vi "001_TCPTransfer.vi"(11 "Queue Ref":T1={"UI"=refnum, "Message"=refnum, "Data"=refnum, "Caller"=refnum, "Name"="000 Common", "Data Path"=path "D:/NBT/01-Project/02-Processing/NBT-TestPlatform V2/NBT-TestPlatform V2.0.3/Config/NBT/NBT_V1.0.0/Project/0001_HZKD_ST01/00_DataSource/001_PLC/01_PLC", "Class Path"=path "", "SubPanel"=refnum, "Project Name"="", "MNT"="", "Title"="", "Data Source"=refnum, "Queue List"={}, "VI"=refnum, "UE"=refnum}) -> ()   [LabVIEW 2020]
doc: "TCP"
uses:
  Alin/QMH/000 Module Data Type.ctl
  Alin/QMH/Queue Message.ctl
  9999 SubVI/Global/Data Global/SDQ Data Type.ctl
  0007 Controls/005 Data Source Type.ctl
  9999 SubVI/Global/Data Global/Data Global Mode.ctl
  9cf45a25-2d87-4abb-9e44-08fab8a6d34b.vi
panel:
  out "Status":bool
  in  "Port":u16=9090
  in  "Open":bool
  in  "Panel Show":bool
  out "Write Data":string
  out "Read Data":string
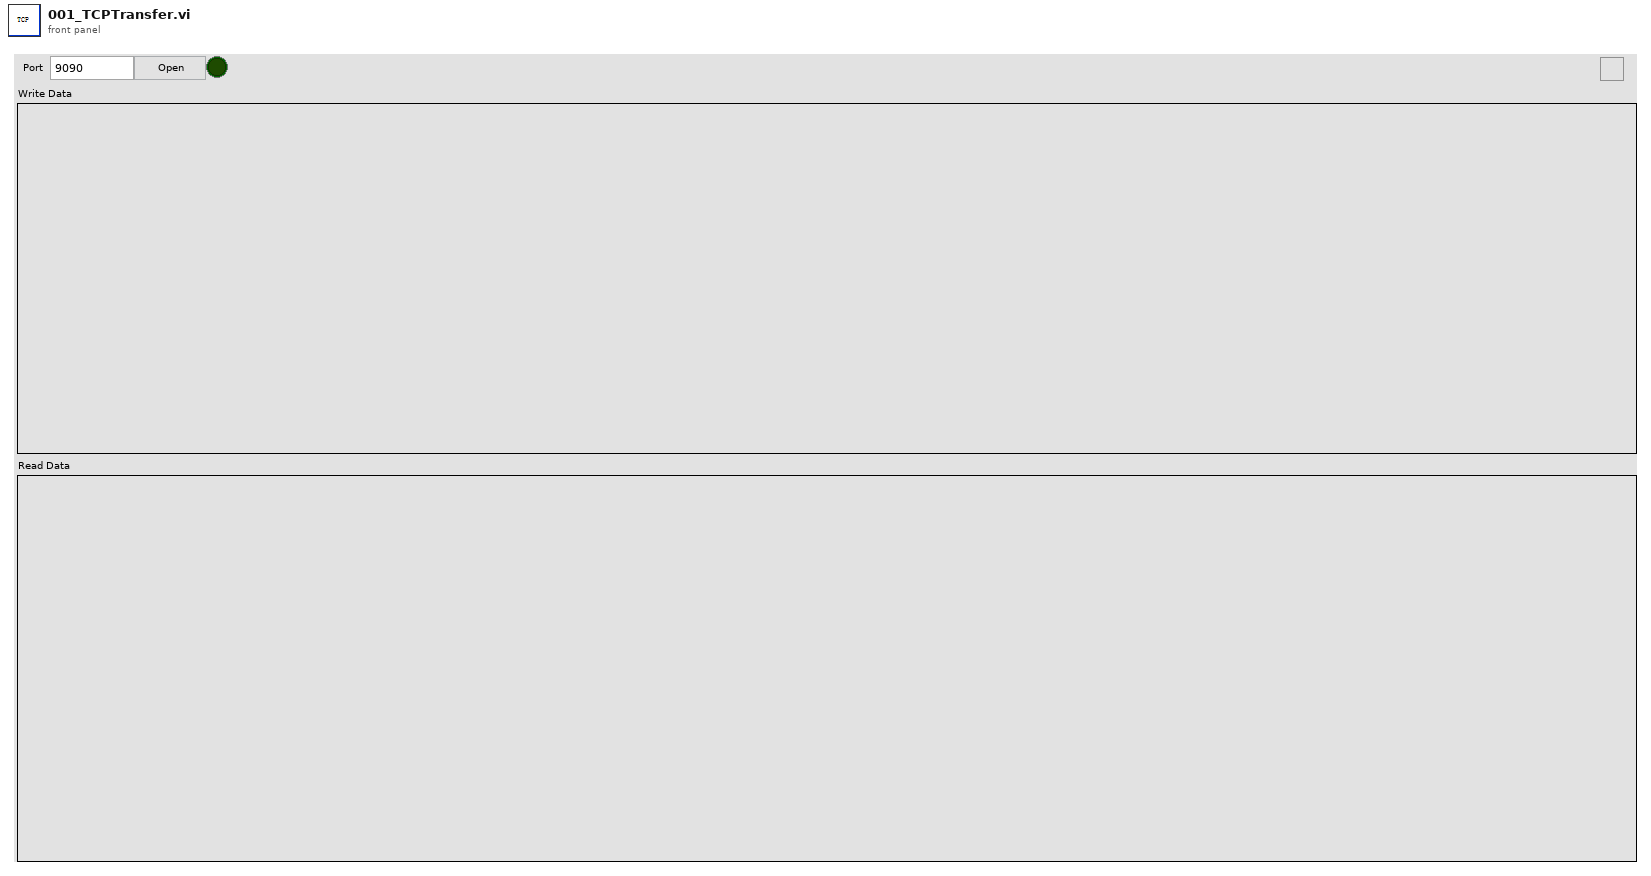
[diagram p1: front panel]
types:
  T1 = typedef "000 Module Data Type.ctl" = cluster{"UI":refnum<queue>, "Message":refnum<queue>, "Data":refnum<queue>, "Caller":refnum<queue>, "Name":string, "Data Path":path, "Class Path":path, "SubPanel":refnum<vi>, "Project Name":string, "MNT":string, "Title":string, "Data Source":refnum<queue>, "Queue List":map{string, refnum<queue>}, "VI":refnum<vi>, "UE":refnum<user-event>}
  T2 = typedef "SDQ Data Type.ctl" = cluster{"CAN Length":string, "CAN Name":string, "CAN ID":string, "CAN Type":string, "Test Item":string, "Byte Order":string, "Instruction":string, "Control Type":string, "Group":string, "Offset":dbl, "Coefficient":dbl, "Write Enable":bool, "Lable Type":string, "Key?":string, "Set Value":string, "Upper":dbl, "Lower":dbl, "Unit":string, "Formula":string, "Test Item Type":string, "Length":i32, "Address":string, "Name":string, "Identifier":string, "Data Type":string, "Enumerate?":string, "Enumerate List":string, "Data":string, "Source":string}
  T3 = typedef "005 Data Source Type.ctl" = cluster{"Device Name":string, "Device Model":string, "Device Driver":string, "IP Address":string, "Port":string, "Remark":string, "Enable":string, "Path":string}
  T4 = cluster{"Read Data":map{string, string}, "Open?":bool, "Start?":bool, "Queue Ref":T1, "Data":map{string, T2}, "Data List":T2[], "Ref":cluster{"Server":refnum<k5>, "Client":refnum<k5>}, "Identifiers":string, "Last Time":u32, "All Data":string[][], "Element":T2, "Title":string[], "Type":map{string, string}, "IP":string, "port":i32, "Next":string, "Data Type Out":T3, "Delay":cluster{"Count Time(ms)":u32, "Delay Time(ms)":u32, "Next":string}}
  T5 = typedef "Data Global Mode.ctl" = enum16{"Init", "Read", "Write", "Write Data", "Load"}
  T6 = cluster{"Server":refnum<k5>, "Client":refnum<k5>}
  T7 = cluster{"Name":string, "Type":map{string, string}}
  T8 = typedef "eventvkey.ctl" = enum16{"ASCII", "Enter", "Return", "Shift", "Ctrl", "Alt", "Cmd", "Opt", "Caps", "NumLock", "Clear", "Break", "Up", "Down", "Left", "Right", "Insert", "Delete", "Home", "End", "PageUp", "PageDown", "Escape", "Help", "Pause", "ScrollLock", "F1", "F2", "F3", "F4", "F5", "F6", "F7", "F8", "F9", "F10", "F11", "F12", "F13", "F14", "F15", "F16", "F17", "F18", "F19", "F20", "F21", "F22", "F23", "F24", "Play", "VolumeUp", "VolumeDown", "Mute", "Two Byte Char"}
  T9 = cluster{"Shift":bool, "Ctrl":bool, "Alt":bool, "Cmd":bool, "Opt":bool}
  T10 = cluster{"Queue List":map{string, refnum<queue>}, "Active Panel":string, "Queue":T1, "Active Row":i32, "All Data":string[][]}
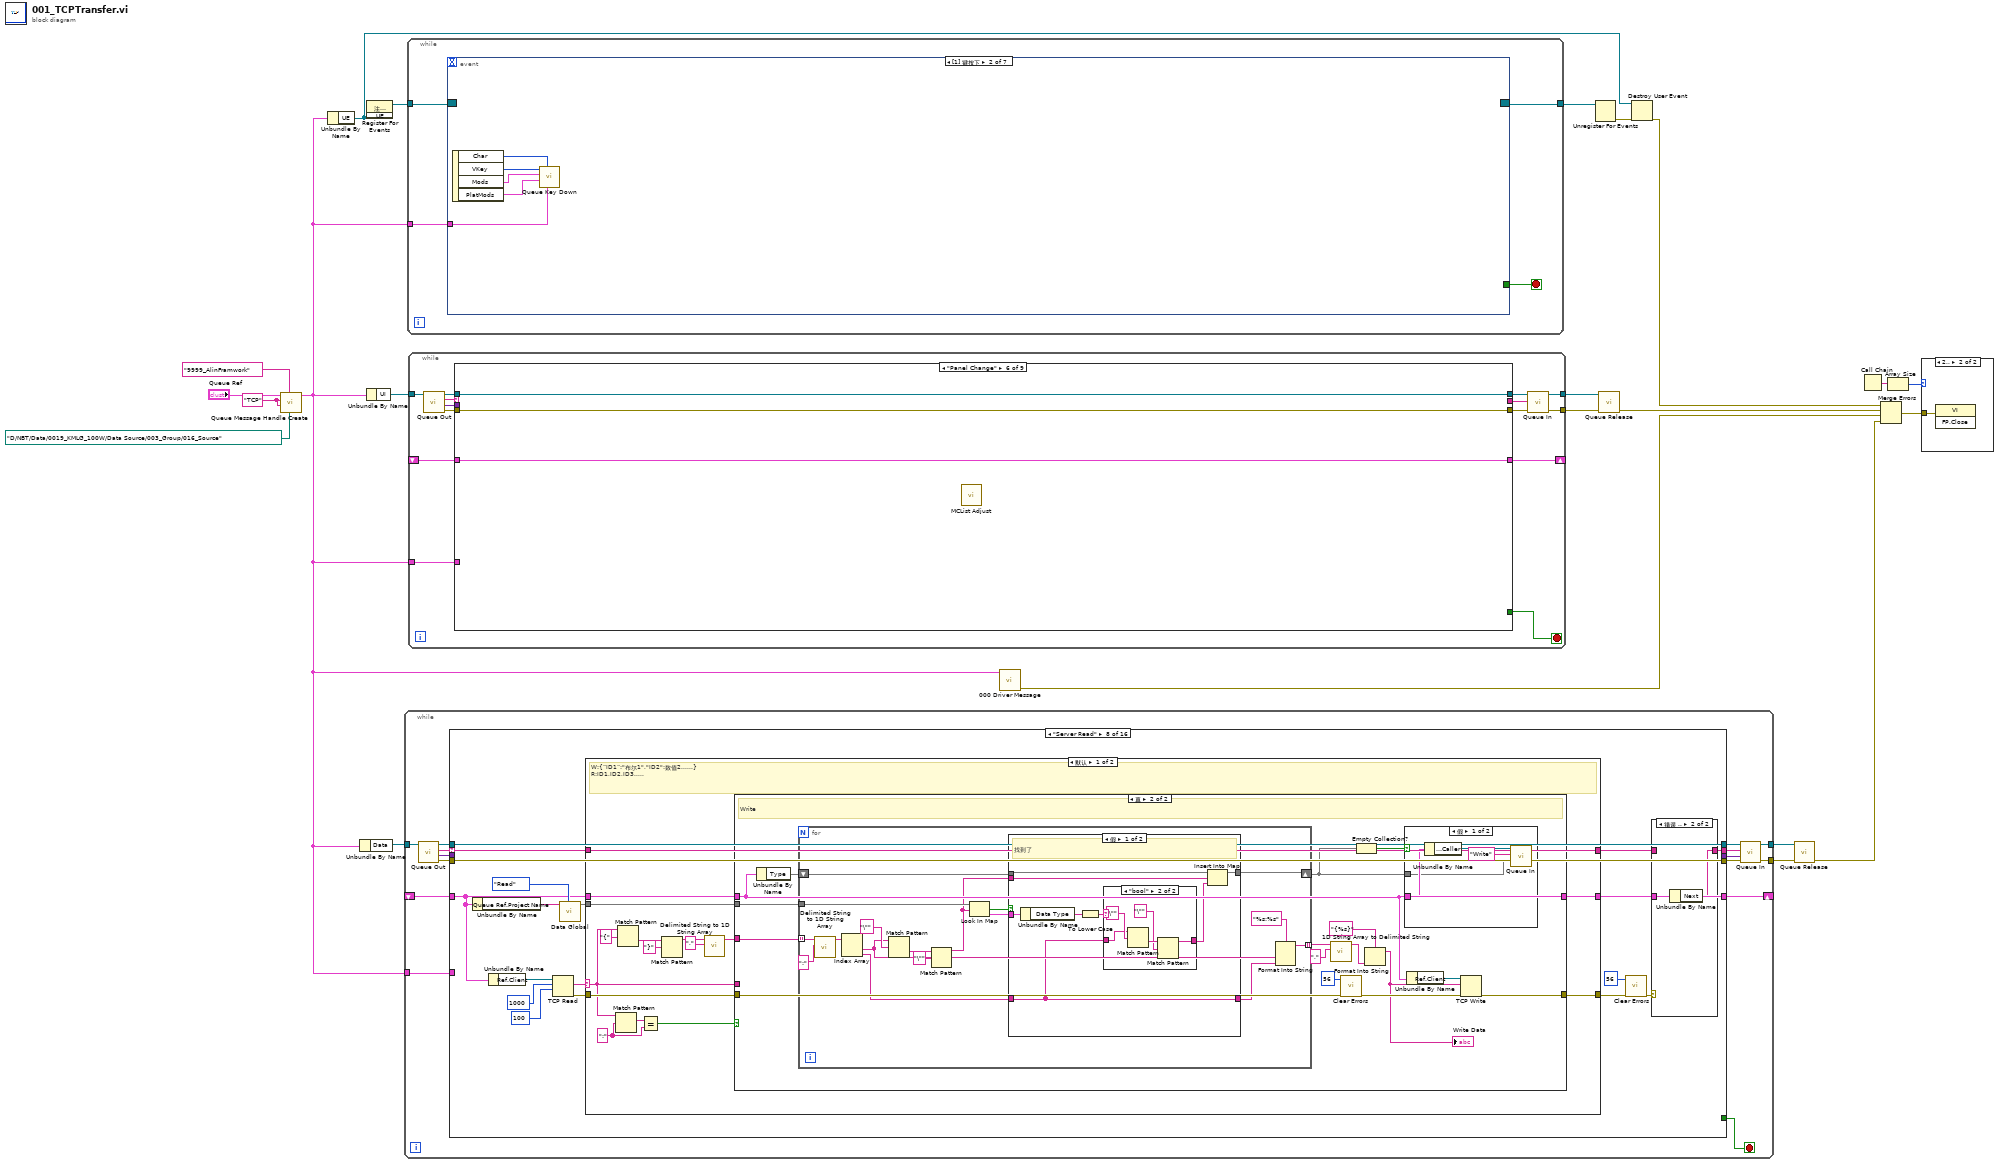
[diagram p0: block diagram]
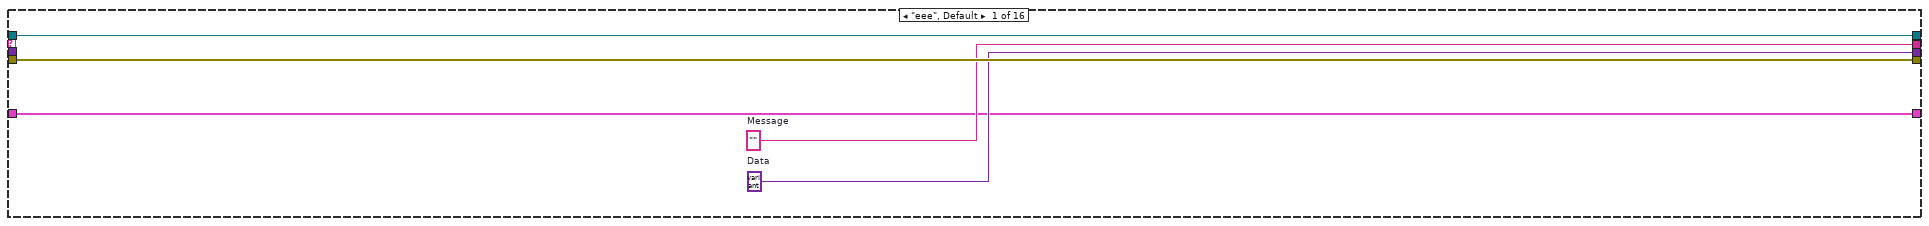
[diagram p2: hidden frame]
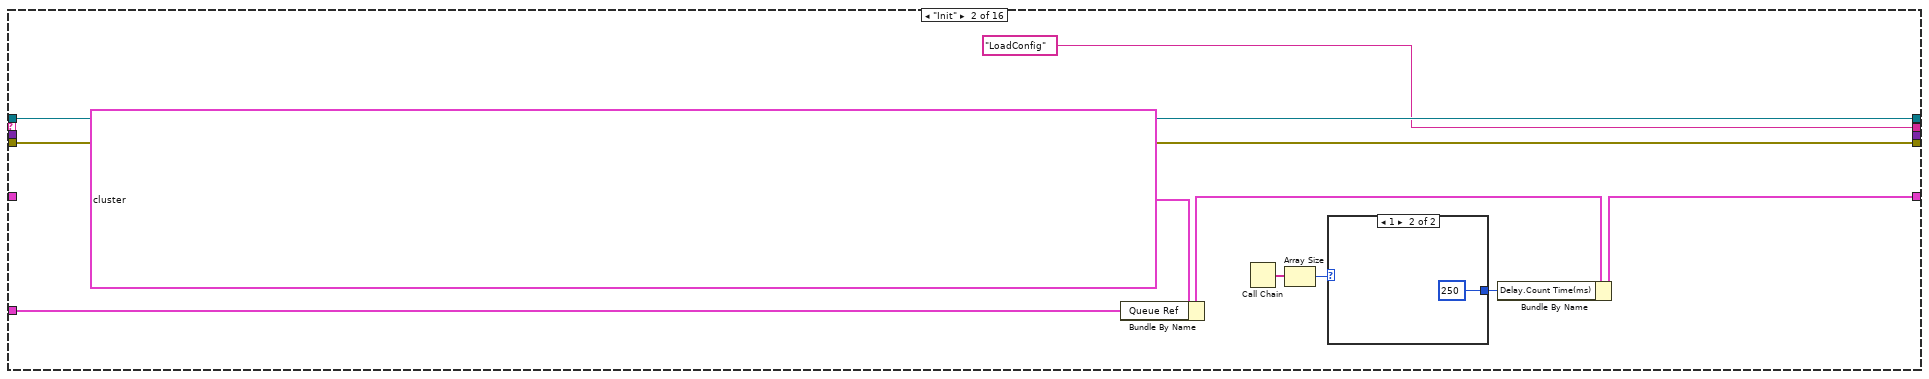
[diagram p3: hidden frame]
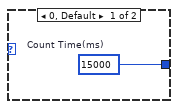
[diagram p4: hidden frame]
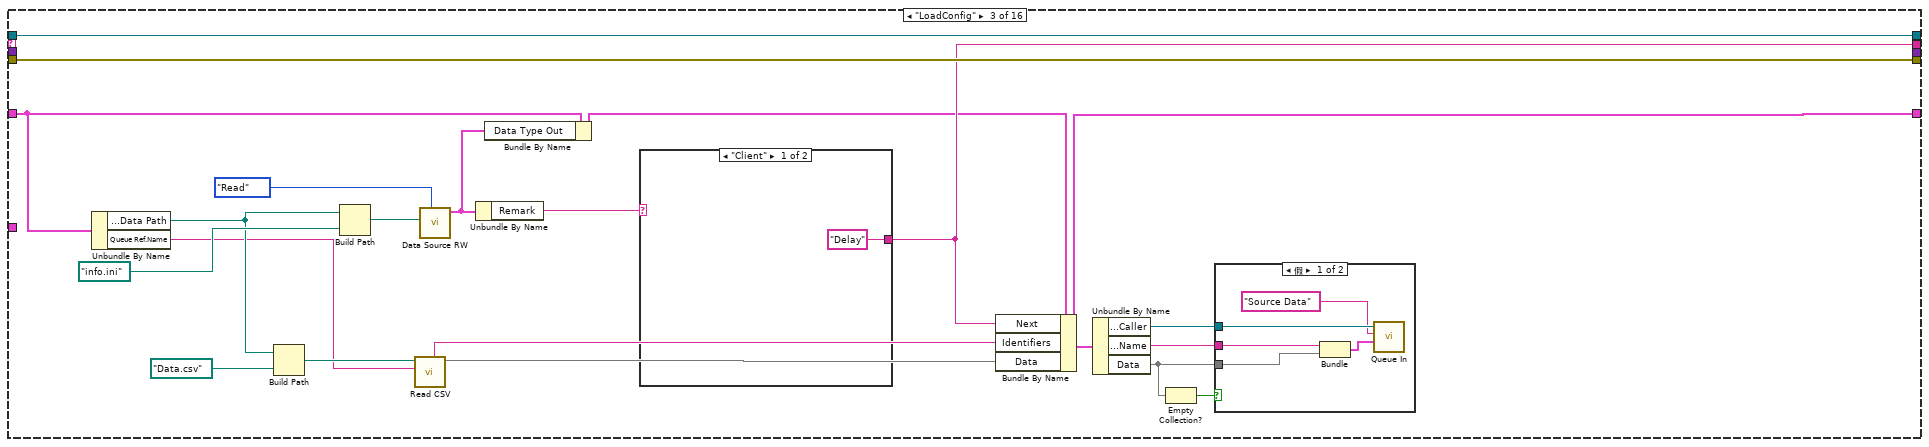
[diagram p5: hidden frame]
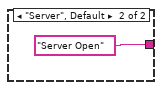
[diagram p7: hidden frame]
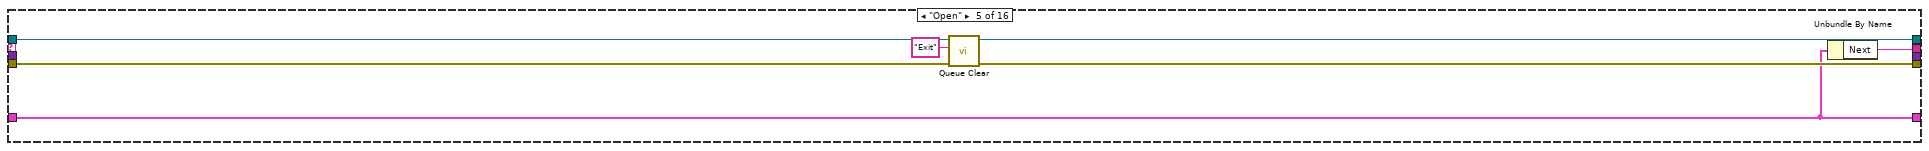
[diagram p9: hidden frame]
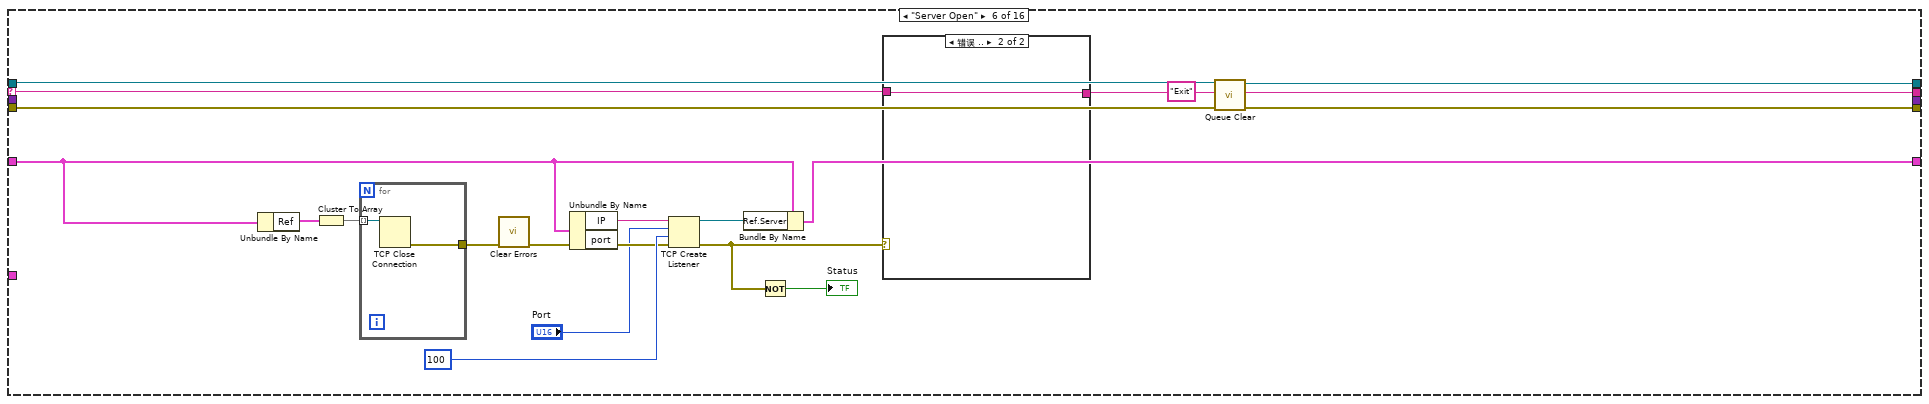
[diagram p10: hidden frame]
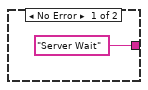
[diagram p11: hidden frame]
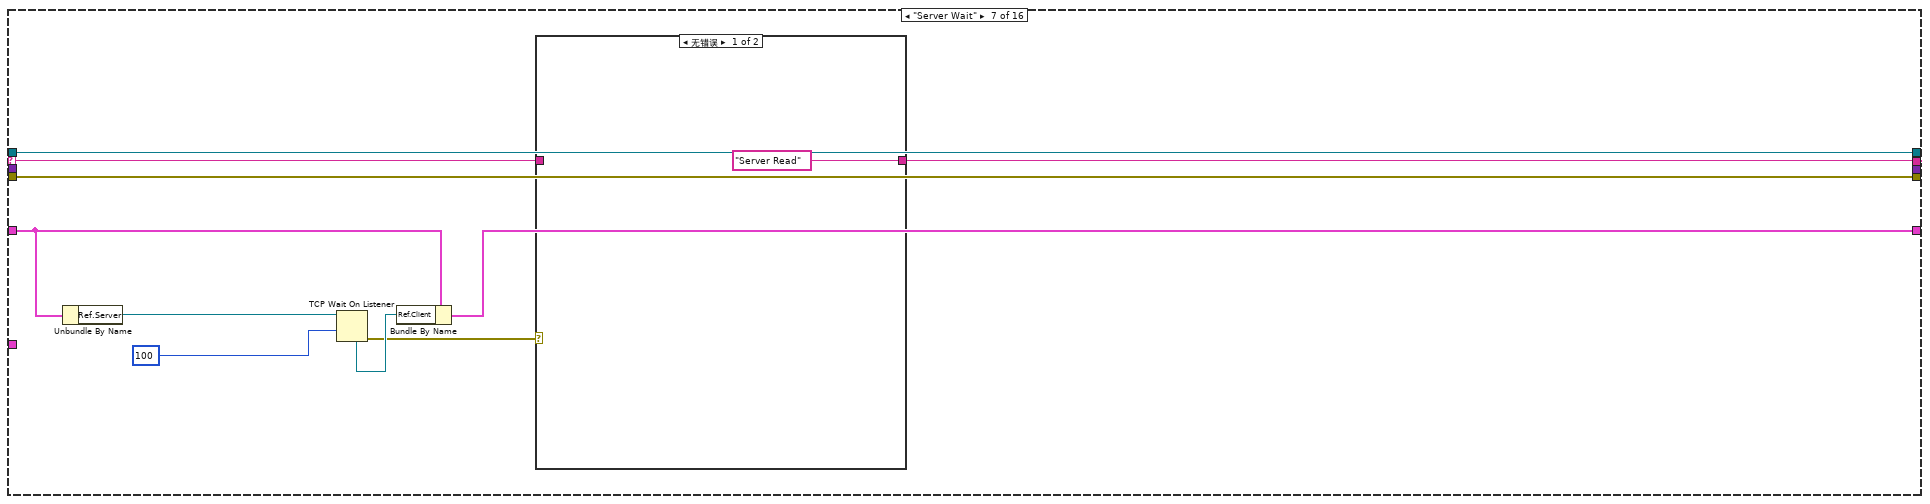
[diagram p12: hidden frame]
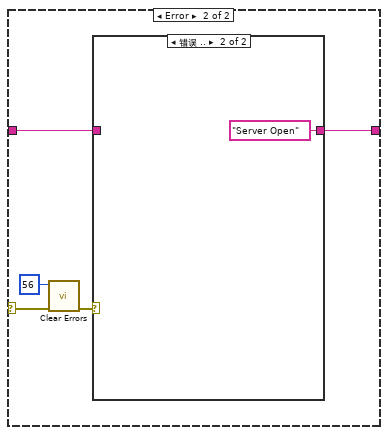
[diagram p13: hidden frame]
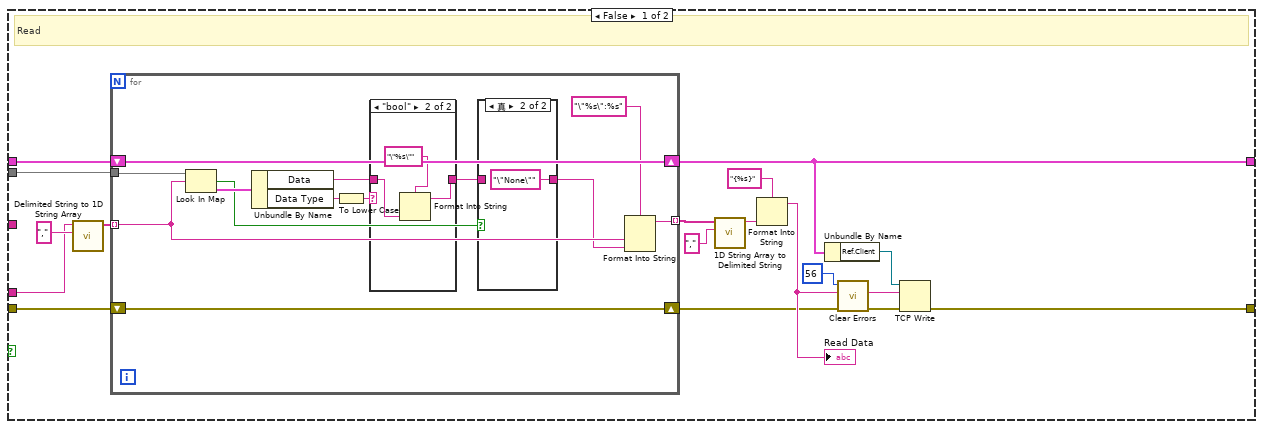
[diagram p16: hidden frame]
diagram:
  w3 = "TCP"
  n1 = call "Queue Message Handle Create.vi"("Data Path"=path "D:/NBT/Data/0019_KMLG_100W/Data Source/003_Group/016_Source", "Project Name"="9999_AlinFramwork", "Name"=w3, "Title"=w3, "Queue Ref In"="Queue Ref") -> ("Queue Ref Out"=w6:T1)  [unwired: 5 in, 1 out]
  n2 = Unbundle By Name(w6) -> ("UE"=w5:refnum<user-event>)
  n3 = Unbundle By Name(w6) -> ("Data"=w20:refnum<queue>)
  n4 = Unbundle By Name(w6) -> ("UI"=w12:refnum<queue>)
  n5 = register-events(w5) -> (reference out=w7:refnum<event-registration>)  [unwired: 2 in, 1 out]
  n6 = while {
    tunnel: w20 -> [w34]
    tunnel: [w31] -> w18
    tunnel: [w30] -> w19
    shift-right: [w24] -> _
    shift-left: _ -> [w26]
    tunnel: w6 -> [w25]
    stop <- w37 stop-if-true
    n7 = call "Queue Out.vi"("Queue In"=w34) -> ("error out"=w36:errorcluster, "Data"=w35:variant, "Message"=w23:string, "Queue Out"=w33:refnum<queue>)  [unwired: 6 in, 1 out]
    n8 = case shown="\"Server Read\"" w23 {
      selector: w23 -> [_ _ _ _ _ w105 w116 w147 w266 w298 w383 _ w428 _ _ _]
      tunnel: w33 -> [w42 w52 w75 w85 w90 w98 w125 w151 w277 w301 w385 w424 w435 w438 w443 w447]
      tunnel: w36 -> [w41 w51 w74 w84 w92 w111 w124 w150 w276 w300 w384 w423 w434 w437 w441 w448]
      tunnel: [w42 w52 w75 w85 w89 w97 w125 w151 w277 w301 w385 w424 w435 w438 w442 w447] -> w32
      tunnel: [w41 w51 w74 w84 w91 w99 w124 w150 w276 w300 w384 w423 w434 w437 w440 w448] -> w29
      tunnel: [w40 "LoadConfig" ("Message") w63 _ w86 w106 w117 w140 w265 w291 w378 _ w427 _ "Close,Quit" _] -> w28
      tunnel: [_ _ _ _ _ _ _ _ _ _ _ _ _ _ _ TRUE] -> w37
      tunnel: [w39 _ _ _ _ _ _ _ _ _ _ _ _ _ _ _] -> w27
      tunnel: w35 -> [_ _ _ _ _ _ _ _ _ _ w375 _ _ _ _ _]
      tunnel: [w38 w44 w58 w83 w87 w107 w120 w134 w268 w286 w376 w422 w429 w436 w439 w445] -> w24
      tunnel: w26 -> [w38 _ w72 w83 w87 w104 w121 w138 w270 w290 w377 w422 w429 w436 w439 w445]
      tunnel: w25 -> [_ w48 _ _ _ _ _ _ _ _ _ _ _ _ _ _]
      frame "eee", Default {
        w39 = variant  # Data
        w40 = ""  # Message
      }
      frame "Init" {
        n9 = Bundle By Name(cluster=T4 {"Read Data"={}, "Open?"=FALSE, "Start?"=FALSE, "Queue Ref"={"UI"=refnum, "Message"=refnum, "Data"=refnum, "Caller"=refnum, "Name"="", "Data Path"=path "", "Class Path"=path "", "SubPanel"=refnum, "Project Name"="", "MNT"="", "Title"="", "Data Source"=refnum, "Queue List"={}, "VI"=refnum, "UE"=refnum}, "Data"={}, "Data List"=[], "Ref"={"Server"=refnum, "Client"=refnum}, "Identifiers"="", "Last Time"=0, "All Data"=[], "Element"={"CAN Length"="", "CAN Name"="", "CAN ID"="", "CAN Type"="", "Test Item"="", "Byte Order"="", "Instruction"="", "Control Type"="", "Group"="", "Offset"=0.0, "Coefficient"=0.0, "Write Enable"=FALSE, "Lable Type"="", "Key?"="", "Set Value"="", "Upper"=0.0, "Lower"=0.0, "Unit"="", "Formula"="", "Test Item Type"="", "Length"=0, "Address"="", "Name"="", "Identifier"="", "Data Type"="", "Enumerate?"="", "Enumerate List"="", "Data"="", "Source"=""}, "Title"=[], "Type"={}, "IP"="127.0.0.1", "port"=4040, "Next"="", "Data Type Out"={"Device Name"="单体电压数据源", "Device Model"="CVM", "Device Driver"="FCTS DAQ", "IP Address"="127.0.0.1", "Port"="8080", "Remark"="CVM读取数据源", "Enable"="False", "Path"="001_Source"}, "Delay"={"Count Time(ms)"=250, "Delay Time(ms)"=250, "Next"="Client Open"}}, "Queue Ref"=w48) -> (w49:T4)
        n10 = Call Chain() -> (call chain=w46:string[])
        n11 = Array Size(array=w46) -> (size(s)=w45:i32)
        n12 = case shown="1" w45 {
          tunnel: [w53 u32 250 ("Count Time(ms)")] -> w43
          frame 0, Default {
            w53 = u32 15000  # Count Time(ms)
          }
          frame 1 {
          }
        }
        n13 = Bundle By Name(cluster=w49, "Delay.Count Time(ms)"=w43) -> (w44:T4)
      }
      frame "LoadConfig" {
        n14 = Unbundle By Name(w72) -> ("Queue Ref.Data Path"=w68:path, "Queue Ref.Name"=w60:string)
        n15 = Build Path(base path=w68, name or relative path=path "Data.csv" ("名称或相对路径")) -> (appended path=w66:path)
        n16 = Build Path(base path=w68, name or relative path=path "info.ini" ("Source Path")) -> (appended path=w70:path)
        n17 = call "Read CSV.vi"("Source"=w60, "Data Path"=w66) -> ("Identifiers Out"=w64:map{string, T2}, "Identifiers"=w65:string)  [unwired: 2 in, 6 out]
        n18 = call "Data Source RW.vi"("Operate"=enum16{"Read", "Write"}."Read", "Source Path"=w70) -> ("Data Type Out"=w62:T3)  [unwired: 6 in, 3 out]
        n19 = Unbundle By Name(w62) -> ("Remark"=w69:string)
        n20 = Bundle By Name(cluster=w72, "Data Type Out"=w62) -> (w61:T4)
        n21 = case shown="\"Client\"" w69 {
          tunnel: ["Delay" "Server Open"] -> w63
          frame "Client" {
          }
          frame "Server", Default {
          }
        }
        n22 = Bundle By Name(cluster=w61, "Next"=w63, "Identifiers"=w65, "Data"=w64) -> (w58:T4)
        n23 = Unbundle By Name(w58) -> ("Queue Ref.Caller"=w59:refnum<queue>, "Queue Ref.Name"=w57:string, "Data"=w56:map{string, T2})
        n24 = Empty Collection?(1:w56) -> (0:w55:bool)
        n25 = case shown="假" w55 {
          tunnel: w59 -> [w80 _]
          tunnel: w57 -> [w78 _]
          tunnel: w56 -> [w76 _]
          frame False {
            n26 = Bundle("Name"=w78, "Data"=w76) -> (w77:cluster{"Name":string, "Data":map{string, T2}})  [unwired: 1 in]
            n27 = call "Queue In.vi"("Data"=w77, "Message"="Source Data", "Queue In"=w80) -> ()  [unwired: 7 in, 2 out]
          }
          frame True {
          }
        }
      }
      frame "====Driver====" {
      }
      frame "Open" {
        n28 = call "Queue Clear.vi"("error in (no error)"=w92, "Filter"="Exit", "Queue In"=w90) -> ("error out"=w91:errorcluster, "Queue Out"=w89:refnum<queue>)  [unwired: 7 in]
        n29 = Unbundle By Name(w87) -> ("Next"=w86:string)
      }
      frame "Server Open" {
        n30 = Unbundle By Name(w104) -> ("Ref"=w103:T6)
        n31 = Cluster To Array(cluster=w103) -> (array=w102:refnum<k5>[])
        n32 = for {
          tunnel: w102 -> [w113] mode=indexing
          tunnel: [w112] -> w101
          n33 = TCP Close Connection(connection ID=w113) -> (error out=w112:errorcluster)  [unwired: 2 in, 1 out]
        }
        n34 = call <vilib>:"Clear Errors.vi"("error in (no error)"=w101) -> ("error out"=w100:errorcluster)  [unwired: 5 in, 1 out]
        n35 = Unbundle By Name(w104) -> ("IP"=w110:string)  [unwired: 1 out]
        n36 = TCP Create Listener(8:w100, 9:100 ("超时毫秒(25000)"), 10:"Port", 11:w110) -> (0:w94:errorcluster, 3:w108:refnum<k5>)  [unwired: 1 in, 1 out]
        n37 = Bundle By Name(cluster=w104, "Ref.Server"=w108) -> (w107:T4)
        n38 = Not(x=w94) -> (.not. x?=→"Status":bool)
        n39 = case shown="错误 .." w94 {
          tunnel: ["Server Wait" w115] -> w106
          tunnel: w105 -> [_ w115]
          frame No Error {
          }
          frame Error {
          }
        }
        n40 = call "Queue Clear.vi"("error in (no error)"=w111, "Filter"="Exit", "Queue In"=w98) -> ("error out"=w99:errorcluster, "Queue Out"=w97:refnum<queue>)  [unwired: 7 in]
      }
      frame "Server Wait" {
        n41 = Unbundle By Name(w121) -> ("Ref.Server"=w123:refnum<k5>)
        n42 = TCP Wait On Listener(9:100 ("超时毫秒（一直等待:-1）"), 11:w123) -> (0:w118:errorcluster, 4:w119:refnum<k5>)  [unwired: 2 in, 3 out]
        n43 = Bundle By Name(cluster=w121, "Ref.Client"=w119) -> (w120:T4)
        n44 = case shown="无错误" w118 {
          selector: w118 -> [_ w131]
          tunnel: ["Server Read" w128] -> w117
          tunnel: w116 -> [_ w127]
          frame No Error {
          }
          frame Error {
            n45 = call <vilib>:"Clear Errors.vi"("error in (no error)"=w131, "specific error code to clear (0: all)"=56) -> ("error out"=w129:errorcluster)  [unwired: 4 in, 1 out]
            n46 = case shown="错误 .." w129 {
              tunnel: [w132 "Server Open"] -> w128
              tunnel: w127 -> [w132 _]
              frame No Error {
              }
              frame Error {
              }
            }
          }
        }
      }
      frame "Server Read" {
        n47 = Unbundle By Name(w138) -> ("Queue Ref.Project Name"=w137:string)
        n48 = Unbundle By Name(w138) -> ("Ref.Client"=w149:refnum<k5>)
        n49 = TCP Read(connection ID=w149, bytes to read=1000 ("读取的字节"), 9:100 ("超时毫秒(25000)")) -> (data out=w145:string, error out=w135:errorcluster)  [unwired: 2 in, 1 out]
        n50 = call "Data Global.vi"("Operate"=Data_Global_Mode."Read", "Name"=w137) -> ("Data Out"=w136:map{string, T2})  [unwired: 6 in, 3 out]
        n51 = case shown="默认" w145 {
          selector: w145 -> [w155 _]
          tunnel: [w159 w262] -> w134
          tunnel: w138 -> [w160 w262]
          tunnel: w147 -> [w170 w261]
          tunnel: [w170 w261] -> w141
          tunnel: [w157 w260] -> w144
          tunnel: w136 -> [w158 _]
          tunnel: w135 -> [w156 w260]
          frame Default {
            w163 = ":" ("正则表达式")
            # "W:{“ID1”:\"布尔1\",\"ID2\":数值2......}\nR:ID1,ID2,ID3....."
            n52 = Match Pattern(string=w155, regular expression=w163) -> (match substring=w164:string)  [unwired: 1 in, 3 out]
            n53 = Match Pattern(string=w155, regular expression="{" ("正则表达式")) -> (after substring=w168:string)  [unwired: 1 in, 3 out]
            n54 = Equal?(x=w164, y=w163) -> (x = y?=w162:bool)
            n55 = Match Pattern(string=w168, regular expression="}" ("正则表达式")) -> (before substring=w166:string)  [unwired: 1 in, 3 out]
            n56 = call <vilib>:"Delimited String to 1D String Array.vi"("delimiter"="," ("delimited string"), "delimited string"=w166) -> ("string array"=w161:string[])  [unwired: 9 in]
            n57 = case shown="真" w162 {
              tunnel: w161 -> [_ w221]
              tunnel: w160 -> [w187 w213]
              tunnel: [w181 w213] -> w159
              tunnel: w158 -> [w186 w220]
              tunnel: [w178 w214] -> w157
              tunnel: w156 -> [w177 w222]
              tunnel: w155 -> [w172 _]
              frame False {
                # "Read"
                n58 = call <vilib>:"Delimited String to 1D String Array.vi"("delimiter"="," ("delimited string"), "delimited string"=w172) -> ("string array"=w171:string[])  [unwired: 9 in]
                n59 = for {
                  tunnel: w171 -> [w200] mode=indexing
                  shift-right: [w199] -> w181
                  shift-left: w187 -> [w199]
                  tunnel: w186 -> [w198]
                  tunnel: [w195] -> w185 mode=indexing
                  shift-right: [w194] -> w176
                  shift-left: w177 -> [w194]
                  n60 = Look In Map(map=w198, key=w200) -> (key not found?=w190:bool, value=w197:T2)  [unwired: 1 in]
                  n61 = Unbundle By Name(w197) -> ("Data"=w191:string, "Data Type"=w193:string)
                  n62 = To Lower Case(string=w193) -> (all lower case string=w192:string)
                  n63 = case shown="\"bool\"" w192 {
                    tunnel: w191 -> [w203 w205]
                    tunnel: [w203 w204] -> w189
                    frame Default {
                    }
                    frame "bool" {
                      n64 = Format Into String(format string="\"%s\"" ("格式字符串"), w205) -> (resulting string=w204:string)  [unwired: 2 in, 1 out]
                    }
                  }
                  n65 = case shown="真" w190 {
                    tunnel: w189 -> [w201 _]
                    tunnel: [w201 "\"None\"" ("Data")] -> w188
                    frame False {
                    }
                    frame True {
                    }
                  }
                  n66 = Format Into String(format string="\"%s\":%s" ("格式字符串"), w200, w188) -> (resulting string=w195:string)  [unwired: 2 in, 1 out]
                }
                n67 = call <vilib>:"1D String Array to Delimited String.vi"("delimiter"=",", "string array"=w185) -> ("delimited string"=w182:string)  [unwired: 9 in]
                n68 = Format Into String(format string="{%s}" ("格式字符串"), w182) -> (resulting string=w179:string)  [unwired: 2 in, 1 out]
                "Read Data" <- w179
                n69 = Unbundle By Name(w181) -> ("Ref.Client"=w180:refnum<k5>)
                n70 = call <vilib>:"Clear Errors.vi"("error in (no error)"=w176, "specific error code to clear (0: all)"=56) -> ("error out"=w175:errorcluster)  [unwired: 4 in, 1 out]
                n71 = TCP Write(connection ID=w180, data in=w179, error in (no error)=w175) -> (error out=w178:errorcluster)  [unwired: 1 in, 2 out]
              }
              frame True {
                # "Write"
                n72 = Unbundle By Name(w213) -> ("Type"=w219:map{string, string})
                n73 = for {
                  tunnel: w221 -> [w242] mode=indexing
                  tunnel: w220 -> [w241]
                  shift-right: [w238] -> w218
                  shift-left: w219 -> [w239]
                  tunnel: [w227] -> w210 mode=indexing
                  n74 = call <vilib>:"Delimited String to 1D String Array.vi"("delimiter"=":" ("delimited string"), "delimited string"=w242) -> ("string array"=w234:string[])  [unwired: 9 in]
                  n75 = Index Array(array=w234) -> (element #1=w229:string, element #2=w233:string)  [unwired: 2 in]
                  n76 = Match Pattern(string=w229, regular expression="\"" ("正则表达式")) -> (after substring=w236:string)  [unwired: 1 in, 3 out]
                  n77 = Match Pattern(string=w236, regular expression="\"" ("正则表达式")) -> (before substring=w231:string)  [unwired: 1 in, 3 out]
                  n78 = Look In Map(map=w241, key=w231) -> (key not found?=w240:bool, value=w232:T2)  [unwired: 1 in]
                  n79 = case shown="假" w240 {
                    tunnel: w239 -> [w251 w259]
                    tunnel: [w250 w259] -> w238
                    tunnel: w233 -> [w244 _]
                    tunnel: w232 -> [w249 _]
                    tunnel: w231 -> [w245 _]
                    tunnel: [w244 "\"None\"" ("String")] -> w228
                    frame False {
                      # "找到了"
                      n80 = Unbundle By Name(w249) -> ("Data Type"=w248:string)
                      n81 = To Lower Case(string=w248) -> (all lower case string=w247:string)
                      n82 = case shown="\"bool\"" w247 {
                        tunnel: w244 -> [w252 w254]
                        tunnel: [w252 w253] -> w246
                        frame Default {
                        }
                        frame "bool" {
                          n83 = Match Pattern(string=w254, regular expression="\"" ("正则表达式")) -> (after substring=w256:string)  [unwired: 1 in, 3 out]
                          n84 = Match Pattern(string=w256, regular expression="\"" ("正则表达式")) -> (before substring=w253:string)  [unwired: 1 in, 3 out]
                        }
                      }
                      n85 = Insert Into Map(map in=w251, key=w245, value=w246) -> (map out=w250:map{string, string})  [unwired: 2 out]
                    }
                    frame True {
                      # "找不到"
                    }
                  }
                  n86 = Format Into String(format string="%s:%s" ("格式字符串"), w229, w228) -> (resulting string=w227:string)  [unwired: 2 in, 1 out]
                }
                n87 = call <vilib>:"1D String Array to Delimited String.vi"("delimiter"=",", "string array"=w210) -> ("delimited string"=w208:string)  [unwired: 9 in]
                n88 = call <vilib>:"Clear Errors.vi"("error in (no error)"=w222, "specific error code to clear (0: all)"=56) -> ("error out"=w215:errorcluster)  [unwired: 4 in, 1 out]
                n89 = Empty Collection?(1:w218) -> (0:w217:bool)
                n90 = Format Into String(format string="{%s}" ("格式字符串"), w208) -> (resulting string=w207:string)  [unwired: 2 in, 1 out]
                "Write Data" <- w207
                n91 = case shown="假" w217 {
                  tunnel: w213 -> [w226 _]
                  tunnel: w218 -> [w225 _]
                  frame False {
                    n92 = Unbundle By Name(w226) -> ("Queue Ref.Caller"=w224:refnum<queue>)
                    n93 = call "Queue In.vi"("Data"=w225, "Message"="Write", "Queue In"=w224) -> ()  [unwired: 7 in, 2 out]
                  }
                  frame True {
                  }
                }
                n94 = Unbundle By Name(w213) -> ("Ref.Client"=w212:refnum<k5>)
                n95 = TCP Write(connection ID=w212, data in=w207, error in (no error)=w215) -> (error out=w214:errorcluster)  [unwired: 1 in, 2 out]
              }
            }
          }
          frame "" {
          }
        }
        n96 = call <vilib>:"Clear Errors.vi"("error in (no error)"=w144, "specific error code to clear (0: all)"=56) -> ("error out"=w142:errorcluster)  [unwired: 4 in, 1 out]
        n97 = case shown="错误 .." w142 {
          tunnel: w141 -> [w152 _]
          tunnel: [w152 w153] -> w140
          tunnel: w134 -> [_ w154]
          frame No Error {
          }
          frame Error {
            n98 = Unbundle By Name(w154) -> ("Next"=w153:string)
          }
        }
      }
      frame "Client Open" {
        n99 = Unbundle By Name(w270) -> ("Ref.Client"=w275:refnum<k5>)
        n100 = TCP Close Connection(connection ID=w275) -> (error out=w274:errorcluster)  [unwired: 2 in, 1 out]
        n101 = call <vilib>:"Clear Errors.vi"("error in (no error)"=w274) -> ("error out"=w273:errorcluster)  [unwired: 5 in, 1 out]
        n102 = local read "Port"() -> (w271:u16)
        n103 = Unbundle By Name(w270) -> ("Data Type Out.IP Address"=w269:string)
        n104 = TCP Open Connection(address=w269, remote port or service name=w271, timeout ms (60000)=100 ("超时毫秒(25000)"), error in (no error)=w273) -> (connection ID=w267:refnum<k5>, error out=w264:errorcluster)  [unwired: 1 in]
        n105 = Bundle By Name(cluster=w270, "Ref.Client"=w267) -> (w268:T4)
        n106 = Not(x=w264) -> (.not. x?=w263:bool)
        n107 = local write "Status"(w263) -> ()
        n108 = case shown="无错误" w264 {
          tunnel: w266 -> [_ w279]
          tunnel: ["Client Read" w279] -> w265
          frame No Error {
          }
          frame Error {
          }
        }
      }
      frame "Client Read" {
        n109 = Unbundle By Name(w290) -> ("Queue Ref.Project Name"=w289:string, "Identifiers"=w280:string)
        n110 = Unbundle By Name(w290) -> ("Ref.Client"=w285:refnum<k5>)
        n111 = TCP Write(connection ID=w285, data in=w280) -> (connection ID out=w283:refnum<k5>, error out=w284:errorcluster)  [unwired: 2 in, 1 out]
        n112 = call "Stall Data Flow.vim"("value in"=w284, "milliseconds to wait"=u32 200) -> ("value out"=w282:errorcluster)  [unwired: 1 out]
        n113 = call "Data Global.vi"("Name"=w289) -> ("Data Out"=w288:map{string, T2})  [unwired: 7 in, 3 out]
        n114 = TCP Read(connection ID=w283, bytes to read=10000 ("读取的字节"), error in (no error)=w282, 9:100 ("超时毫秒(25000)")) -> (data out=w296:string, error out=w287:errorcluster)  [unwired: 1 in, 1 out]
        n115 = case shown="默认" w296 {
          selector: w296 -> [w305 _]
          tunnel: [w313 w370] -> w286
          tunnel: w290 -> [w313 w370]
          tunnel: w298 -> [w320 w369]
          tunnel: [w320 w369] -> w292
          tunnel: [w311 w368] -> w295
          tunnel: w288 -> [w312 _]
          tunnel: w287 -> [w310 w368]
          frame Default {
            # "W:{“ID1”:\"布尔1\",\"ID2\":数值2......}\nR:ID1,ID2,ID3....."
            n116 = local write "Read Data"(w305) -> ()
            n117 = Match Pattern(string=w305, regular expression="{" ("正则表达式")) -> (after substring=w318:string)  [unwired: 1 in, 3 out]
            n118 = Unbundle By Name(w313) -> ("Type"=w309:map{string, string})
            n119 = Match Pattern(string=w318, regular expression="}" ("正则表达式")) -> (before substring=w316:string)  [unwired: 1 in, 3 out]
            n120 = call <vilib>:"Delimited String to 1D String Array.vi"("delimiter"="," ("delimited string"), "delimited string"=w316) -> ("string array"=w314:string[])  [unwired: 9 in]
            n121 = for {
              tunnel: w314 -> [w342] mode=indexing
              tunnel: w312 -> [w341]
              shift-right: [w339] -> w308
              shift-left: w309 -> [w340]
              n122 = call <vilib>:"Delimited String to 1D String Array.vi"("delimiter"=":" ("delimited string"), "delimited string"=w342) -> ("string array"=w335:string[])  [unwired: 9 in]
              n123 = Index Array(array=w335) -> (element #1=w331:string, element #2=w334:string)  [unwired: 2 in]
              n124 = Match Pattern(string=w331, regular expression="\"" ("正则表达式")) -> (after substring=w337:string)  [unwired: 1 in, 3 out]
              n125 = Match Pattern(string=w337, regular expression="\"" ("正则表达式")) -> (before substring=w332:string)  [unwired: 1 in, 3 out]
              n126 = Look In Map(map=w341, key=w332) -> (value=w333:T2)  [unwired: 1 in, 1 out]
              n127 = Unbundle By Name(w333) -> ("Data Type"=w330:string)
              n128 = To Lower Case(string=w330) -> (all lower case string=w329:string)
              n129 = case shown="默认" w329 {
                tunnel: w334 -> [w362 w364]
                tunnel: [w362 w363] -> w328
                frame Default {
                }
                frame "bool" {
                  n130 = Match Pattern(string=w364, regular expression="\"" ("正则表达式")) -> (after substring=w366:string)  [unwired: 1 in, 3 out]
                  n131 = Match Pattern(string=w366, regular expression="\"" ("正则表达式")) -> (before substring=w363:string)  [unwired: 1 in, 3 out]
                }
              }
              n132 = case shown="默认" w332 {
                selector: w332 -> [w347 _]
                tunnel: w340 -> [w349 w361]
                tunnel: [w348 w361] -> w339
                tunnel: w328 -> [w346 _]
                tunnel: "\"None\"" ("y") -> [w345 _]
                frame Default {
                  n133 = Equal?(x=w346, y=w345) -> (x = y?=w344:bool)
                  n134 = case shown="默认" w346 {
                    selector: w346 -> [w351 _]
                    tunnel: w349 -> [w354 w360]
                    tunnel: [w353 w360] -> w348
                    tunnel: w347 -> [w352 _]
                    tunnel: w344 -> [w350 _]
                    frame Default {
                      n135 = case shown="真" w350 {
                        tunnel: w354 -> [w358 w359]
                        tunnel: [w357 w359] -> w353
                        tunnel: w352 -> [w356 _]
                        tunnel: w351 -> [w355 _]
                        frame False {
                          n136 = Insert Into Map(map in=w358, key=w356, value=w355) -> (map out=w357:map{string, string})  [unwired: 2 out]
                        }
                        frame True {
                        }
                      }
                    }
                    frame "", "None" {
                    }
                  }
                }
                frame "" {
                }
              }
            }
            n137 = call <vilib>:"Clear Errors.vi"("error in (no error)"=w310, "specific error code to clear (0: all)"=56) -> ("error out"=w311:errorcluster)  [unwired: 4 in, 1 out]
            n138 = Empty Collection?(1:w308) -> (0:w307:bool)
            n139 = case shown="假" w307 {
              tunnel: w313 -> [w326 _]
              tunnel: w308 -> [w323 _]
              frame False {
                n140 = Unbundle By Name(w326) -> ("Queue Ref.Caller"=w325:refnum<queue>, "Queue Ref.Name"=w322:string)
                n141 = Bundle("Name"=w322, "Type"=w323) -> (w321:T7)  [unwired: 1 in]
                n142 = call "Queue In.vi"("Data"=w321, "Message"="Read", "Queue In"=w325) -> ()  [unwired: 7 in, 2 out]
              }
              frame True {
              }
            }
          }
          frame "" {
          }
        }
        n143 = call <vilib>:"Clear Errors.vi"("error in (no error)"=w295, "specific error code to clear (0: all)"=56) -> ("error out"=w293:errorcluster)  [unwired: 4 in, 1 out]
        n144 = case shown="无错误" w293 {
          tunnel: w292 -> [w302 _]
          tunnel: [w302 w303] -> w291
          tunnel: w286 -> [_ w304]
          frame No Error {
          }
          frame Error {
            n145 = Unbundle By Name(w304) -> ("Next"=w303:string)
          }
        }
      }
      frame "Write" {
        n146 = Unbundle By Name(w377) -> ("Data"=w371:map{string, T2}, "Type"=w374:map{string, string})
        n147 = Variant To Data(type=w374, Variant=w375) -> (data=w373:map{string, string}, error out=w372:errorcluster)  [unwired: 1 in]
        n148 = case shown="无错误" w372 {
          tunnel: [w398 w417] -> w376
          tunnel: w377 -> [w398 w417]
          tunnel: w383 -> [w399 w416]
          tunnel: [w399 w416] -> w379
          tunnel: [w397 _] -> w382
          tunnel: w373 -> [w391 _]
          tunnel: w371 -> [w390 _]
          frame No Error {
            # "W:{“ID1”:\"布尔1\",\"ID2\":数值2......}\nR:ID1,ID2,ID3....."
            n149 = for {
              tunnel: w391 -> [w406] mode=indexing
              tunnel: [w407] -> w394 mode=indexing
              tunnel: w390 -> [w404]
              n150 = Unbundle By Name(w406) -> ("Identifier"=w403:string, "Data"=w405:string)
              n151 = Look In Map(map=w404, key=w403) -> (value=w402:T2)  [unwired: 1 in, 1 out]
              n152 = Unbundle By Name(w402) -> ("Data Type"=w401:string)
              n153 = To Lower Case(string=w401) -> (all lower case string=w400:string)
              n154 = case shown="默认" w400 {
                tunnel: [w410 w412] -> w407
                tunnel: w405 -> [w409 w414]
                tunnel: w403 -> [w408 w413]
                frame Default {
                  n155 = Format Into String(format string="\"%s\":%s" ("格式字符串"), w408, w409) -> (resulting string=w410:string)  [unwired: 2 in, 1 out]
                }
                frame "bool" {
                  n156 = Format Into String(format string="\"%s\":\"%s\"" ("格式字符串"), w413, w414) -> (resulting string=w412:string)  [unwired: 2 in, 1 out]
                }
              }
            }
            n157 = call <vilib>:"1D String Array to Delimited String.vi"("delimiter"=",", "string array"=w394) -> ("delimited string"=w392:string)  [unwired: 9 in]
            n158 = Format Into String(format string="{%s}" ("格式字符串"), w392) -> (resulting string=w389:string)  [unwired: 2 in, 1 out]
            n159 = Unbundle By Name(w398) -> ("Ref.Client"=w396:refnum<k5>)
            n160 = local write "Write Data"(w389) -> ()
            n161 = TCP Write ("写入TCP数据")(connection ID=w396, data in=w389) -> (error out=w397:errorcluster)  [unwired: 2 in, 2 out]
          }
          frame Error {
          }
        }
        n162 = call <vilib>:"Clear Errors.vi"("error in (no error)"=w382, "specific error code to clear (0: all)"=56) -> ("error out"=w380:errorcluster)  [unwired: 4 in, 1 out]
        n163 = case shown="错误 .." w380 {
          tunnel: w379 -> [w386 _]
          tunnel: [w386 w387] -> w378
          tunnel: w376 -> [_ w388]
          frame No Error {
          }
          frame Error {
            n164 = Unbundle By Name(w388) -> ("Next"=w387:string)
          }
        }
      }
      frame "Close" {
        n165 = Unbundle By Name(w422) -> ("Ref.Server"=w421:refnum<k5>, "Ref.Client"=w420:refnum<k5>)
        n166 = Build Array(w421, w420) -> (w419:refnum<k5>[])
        n167 = for {
          tunnel: w419 -> [w426] mode=indexing
          tunnel: [w425] -> w418
          n168 = TCP Close Connection(connection ID=w426) -> (error out=w425:errorcluster)  [unwired: 2 in, 1 out]
        }
        n169 = call <vilib>:"Clear Errors.vi"("error in (no error)"=w418) -> ()  [unwired: 5 in, 2 out]
      }
      frame "Delay" {
        n170 = Unbundle By Name(w429) -> ("Delay.Next"=w433:string, "Delay.Count Time(ms)"=w430:u32, "Delay.Delay Time(ms)"=w431:u32)
        n171 = call "Delay Judge.vi"("Delay Time(ms)"=w431, "Count Time(ms)"=w430) -> ("Time Out?"=w432:bool)  [unwired: 5 in, 4 out]
        n172 = Select(t=w433, s=w432, f=w428) -> (s? t:f=w427:string)
      }
      frame "====system====" {
      }
      frame "Exit" {
        n173 = call "Queue Clear.vi"("error in (no error)"=w441, "Queue In"=w443) -> ("error out"=w440:errorcluster, "Queue Out"=w442:refnum<queue>)  [unwired: 8 in]
      }
      frame "Quit" {
      }
    }
    n174 = call "Queue In.vi"("error in (no error)"=w29, "Data"=w27, "Message"=w28, "Queue In"=w32) -> ("error out"=w30:errorcluster, "Queue Out"=w31:refnum<queue>)  [unwired: 6 in]
  }
  n175 = while {
    tunnel: w7 -> [w452]
    tunnel: [w450] -> w8
    tunnel: w6 -> [w449]
    stop <- w451 stop-if-true
    n176 = event shown="[1] 键按下" {
      selector: w452 -> [_ _ _ _ _ _ _]
      dyn-events: [_ _ _ _ _ _ _] -> w450
      timeout: _ -> [_ _ _ _ _ _ _]
      tunnel: [_ _ _ _ w465 _ _] -> w451
      tunnel: w449 -> [_ w457 w461 w464 _ w469 w478]
      event Timeout {
        n177 = event-data() -> ()  [unwired: 1 in, 1 out]
      }
      event Key Down {
        n178 = event-data() -> ("Char"=w456:i16, "VKey"=w455:T8, "Mods"=w454:cluster{"Num Pad":bool, "Menu Key":bool}, "PlatMods"=w453:T9)  [unwired: 1 in]
        n179 = call "Queue Key Down.vi"("Queue Ref Out"=w457, "C"=w456, "Platform Key"=w453, "Group Key"=w454, "V Key"=w455) -> ()  [unwired: 6 in, 1 out]
      }
      event "Panel Show": Value Change {
        n180 = event-data() -> ("CtlRef"=w459:refnum<vi>)  [unwired: 1 in]
        n181 = Unbundle By Name(w461) -> ("Message"=w460:refnum<queue>)
        n182 = property class="Bool"(reference=w459) -> ("Label.Text"=w458:string)  [unwired: 1 in, 2 out]
        n183 = call "Queue In.vi"("Message"=w458, "Queue In"=w460) -> ()  [unwired: 8 in, 2 out]
      }
      event Panel Resize {
        n184 = event-data() -> ()  [unwired: 1 in, 1 out]
        n185 = Unbundle By Name(w464) -> ("Message"=w463:refnum<queue>)
        n186 = call "Queue In.vi"("Message"="Panel Change", "Queue In"=w463) -> ()  [unwired: 8 in, 2 out]
      }
      event User Event {
        n187 = event-data() -> ("Message"=w467:string)  [unwired: 1 in]
        n188 = Equal?(x=w467, y="Exit") -> (x = y?=w465:bool)
      }
      event Panel Close? {
        n189 = event-data() -> ()  [unwired: 1 in, 1 out]
        n190 = Unbundle By Name(w469) -> ("Message"=w468:refnum<queue>)
        n191 = Call Chain() -> (call chain=w472:string[])
        n192 = Array Size(array=w472) -> (size(s)=w471:i32)
        n193 = case shown="0, 默认" w471 {
          tunnel: ["Exit Prepare" ("Message") "Panel Hidden" ("Message")] -> w470
          frame 0, Default {
          }
          frame 2.. {
          }
        }
        n194 = call "Queue In.vi"("Message"=w470, "Queue In"=w468) -> ()  [unwired: 8 in, 2 out]
        n195 = event-data("Discard?"=TRUE ("放弃？")) -> ()  [unwired: 1 in, 1 out]
      }
      event "Open": Value Change {
        n196 = event-data() -> ()  [unwired: 1 in, 1 out]
        n197 = Unbundle By Name(w478) -> ("Data"=w477:refnum<queue>)
        n198 = call "Queue In.vi"("Message"="Open", "Queue In"=w477) -> ()  [unwired: 8 in, 2 out]
      }
    }
  }
  n199 = while {
    tunnel: w12 -> [w488]
    tunnel: [w485] -> w10
    tunnel: [w484] -> w11
    tunnel: w6 -> [w481]
    shift-right: [w480] -> _
    shift-left: _ -> [w479]
    stop <- w492 stop-if-true
    n200 = call "Queue Out.vi"("Queue In"=w488) -> ("error out"=w491:errorcluster, "Data"=w489:variant, "Message"=w490:string, "Queue Out"=w487:refnum<queue>)  [unwired: 6 in, 1 out]
    n201 = case shown="\"Panel Change\"" w490 {
      selector: w490 -> [_ _ _ _ _ _ _ w528 _]
      tunnel: w487 -> [w495 w501 w505 w513 w519 w522 w525 w535 w542]
      tunnel: w491 -> [w494 w500 w504 w512 w518 w521 w524 w533 w543]
      tunnel: [w495 w501 w505 w513 w519 w522 w525 w534 w542] -> w486
      tunnel: [w494 w500 w504 w512 w518 w521 w524 w532 w543] -> w483
      tunnel: [_ "Panel Change" _ _ _ _ _ "Quit" _] -> w482
      tunnel: [_ _ _ _ _ _ _ _ TRUE] -> w492
      tunnel: w489 -> [_ _ w502 w509 _ _ _ _ _]
      tunnel: w481 -> [_ w496 _ _ _ _ _ _ _]
      tunnel: [w493 w497 w503 w510 w517 w520 w523 w527 w540] -> w480
      tunnel: w479 -> [w493 _ w503 w511 w517 w520 w523 w527 w540]
      frame "eee", Default {
      }
      frame "Init" {
        n202 = Bundle By Name(cluster=T10 {"Queue List"={}, "Active Panel"="", "Queue"={"UI"=refnum, "Message"=refnum, "Data"=refnum, "Caller"=refnum, "Name"="", "Data Path"=path "", "Class Path"=path "", "SubPanel"=refnum, "Project Name"="", "MNT"="", "Title"="", "Data Source"=refnum, "Queue List"={}, "VI"=refnum, "UE"=refnum}, "Active Row"=0, "All Data"=[]}, "Queue"=w496) -> (w497:T10)
      }
      frame "Refresh Class Ref" {
        n203 = in-place {
          in-place-border: w502 -> [w508]
          n204 = in-place-cluster #1(w503) -> ("Queue"=w507:T1)
          n205 = Variant To Data(type=w507, Variant=w508) -> (data=w506:T1)  [unwired: 1 in, 1 out]
          n206 = in-place-cluster #1("Queue"=w506) -> ()  [unwired: 1 out]
        }
      }
      frame "Data Change" {
        n207 = in-place {
          in-place-border: w509 -> [w516]
          n208 = in-place-cluster #2(w511) -> ("All Data"=w515:string[][])
          n209 = Variant To Data(type=w515, Variant=w516) -> (data=w514:string[][])  [unwired: 1 in, 1 out]
          n210 = in-place-cluster #2("All Data"=w514) -> (w510:T10)
        }
      }
      frame "====System====" {
      }
      frame "Panel Change" {
        n211 = call "MCList Adjust.vi"() -> ()  [unwired: 11 in, 1 out]
      }
      frame "====User====" {
      }
      frame "Exit" {
        n212 = Unbundle By Name(w527) -> ("Queue.UE"=w526:refnum<user-event>, "Queue.Message"=w531:refnum<queue>, "Queue.Data"=w530:refnum<queue>)
        n213 = Build Array(w531, w530) -> (w529:refnum<queue>[])
        n214 = for {
          tunnel: w529 -> [w539] mode=indexing
          tunnel: w528 -> [w538]
          n215 = call "Queue In.vi"("First"=TRUE, "Message"=w538, "Queue In"=w539) -> ()  [unwired: 7 in, 2 out]
        }
        n216 = Generate User Event(user event=w526, event data cluster=w528) -> ()  [unwired: 2 in, 2 out]
        n217 = call "Queue Clear.vi"("error in (no error)"=w533, "Queue In"=w535) -> ("error out"=w532:errorcluster, "Queue Out"=w534:refnum<queue>)  [unwired: 8 in]
      }
      frame "Quit" {
      }
    }
    n218 = call "Queue In.vi"("error in (no error)"=w483, "Message"=w482, "Queue In"=w486) -> ("error out"=w484:errorcluster, "Queue Out"=w485:refnum<queue>)  [unwired: 7 in]
  }
  n219 = call "000 Driver Message.vi"("Queue In"=w6) -> ("error out"=w21:errorcluster)  [unwired: 8 in, 2 out]
  n220 = Unregister For Events(event registration refnum=w8) -> (error out=w9:errorcluster)  [unwired: 1 in]
  n221 = call "Queue Release.vi"("error in (no error)"=w11, "Queue In"=w10) -> ("error out"=w14:errorcluster)  [unwired: 9 in]
  n222 = Destroy User Event(user event=w5, error in=w9) -> (error out=w13:errorcluster)
  n223 = call "Queue Release.vi"("error in (no error)"=w19, "Queue In"=w18) -> ("error out"=w22:errorcluster)  [unwired: 9 in]
  n224 = Call Chain() -> (call chain=w16:string[])
  n225 = Merge Errors(w13, w14, w21, w22) -> (w15:errorcluster)
  n226 = Array Size(array=w16) -> (size(s)=w17:i32)
  n227 = case shown="2.." w17 {
    tunnel: w15 -> [_ w544]
    frame 0, Default {
    }
    frame 2.. {
      n228 = invoke class="VI" method="FP.Close"(error in=w544) -> ()  [unwired: 2 in, 3 out]
    }
  }
